vi "IMAQ_SUM_Bella.vi"(11 "Image":T1) -> (1 "empty Image":bool, 2 "Sum":sgl, 3 "Image out":T1)   [LabVIEW 2020]
uses:
  IMAQ Image.ctl
  NI_Vision_Development_Module.lvlib
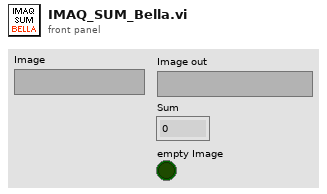
[diagram p1: front panel]
types:
  T1 = typedef "IMAQ Image.ctl" = refnum<image>
  T2 = cluster{"histogram":u32[], "Minimal Value":sgl, "Maximal Value":sgl, "Starting Value":sgl, "Interval Width":sgl, "Mean Value":sgl, "Standard  Variation":sgl, "Area (pixels)":i32}
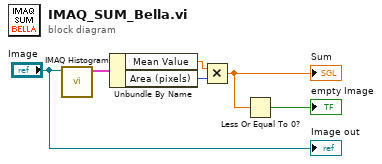
[diagram p0: block diagram]
diagram:
  n1 = call "IMAQ Histogram"("Image"="Image") -> ("Histogram Report"=w6:T2)  [unwired: 9 in, 1 out]
  n2 = Unbundle By Name(w6) -> ("Mean Value"=w5:sgl, "Area (pixels)"=w4:i32)
  n3 = Multiply(x=w5, y=w4) -> (x*y=w2:sgl)
  "Sum" <- w2
  n4 = Less Or Equal To 0?(x=w2) -> (x <= 0?=→"empty Image":bool)
  "Image out" <- "Image"
